vi "Read Given Name.vi"(11 "Attribute.Identity in":refnum<class "Attribute.Identity.lvclass">) -> (2 "Given Name":string, 3 "Attribute.Identity out":refnum<class "Attribute.Identity.lvclass">)   [LabVIEW 2013, in "Attribute.Identity.lvclass"]
uses:
  Attribute.Identity.lvclass
  Attribute.Identity.lvclass/Attribute.Identity.ctl
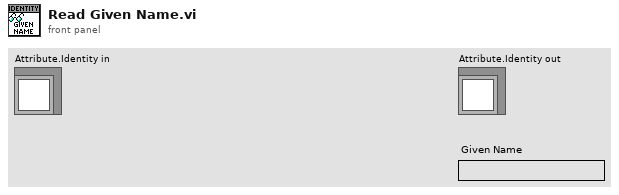
[diagram p1: front panel]
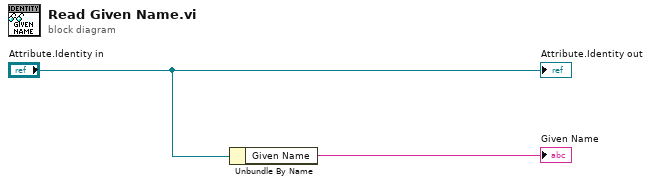
[diagram p0: block diagram]
diagram:
  n1 = Unbundle By Name("Attribute.Identity in") -> ("Given Name"=→"Given Name":string)
  "Attribute.Identity out" <- "Attribute.Identity in"
